vi "GetCalcEveryScanPar.vi"(8 "error in (no error)":errorcluster, 11 "Calculations in":refnum<class "Calculations.lvclass">) -> (0 "error out":errorcluster, 2 "CalcEveryScanPar":bool, 3 "Calculations out":refnum<class "Calculations.lvclass">)   [LabVIEW 2019, in "Calculations.lvclass"]
uses:
  Calculations.lvclass
  Calculations.lvclass/Calculations.ctl
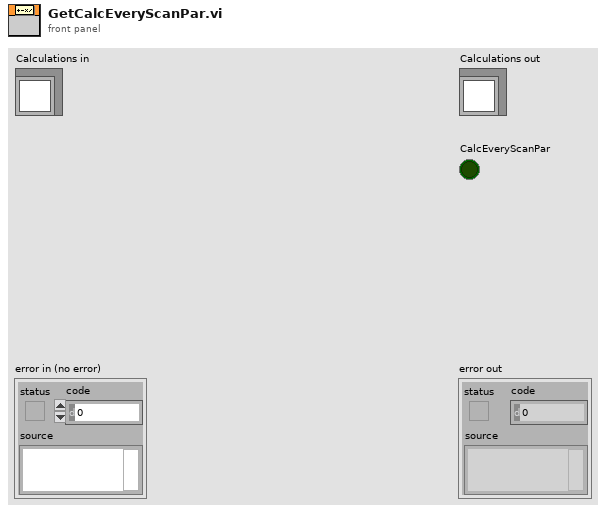
[diagram p1: front panel]
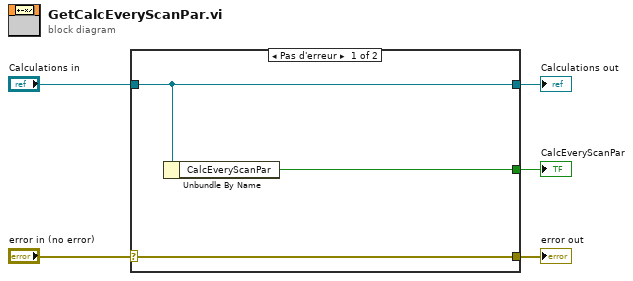
[diagram p0: block diagram]
diagram:
  n1 = case shown="Pas d'erreur" "error in (no error)" {
    selector: "error in (no error)" -> [w8 w9]
    tunnel: [w8 w9] -> w4
    tunnel: [w7 w10] -> w2
    tunnel: "Calculations in" -> [w7 w10]
    tunnel: [w6 _] -> w1
    frame No Error {
      n2 = Unbundle By Name(w7) -> ("CalcEveryScanPar"=w6:bool)
    }
    frame Error {
    }
  }
  "error out" <- w4
  "Calculations out" <- w2
  "CalcEveryScanPar" <- w1
